vi "Main.vi"() -> ()   [LabVIEW 2022 SP3]
panel:
  in  "Number 8":dbl
  out "Result 4":dbl
  in  "Number 7":dbl
  in  "Number 6":dbl
  out "Result 3":dbl
  in  "Number 5":dbl
  in  "Number 4":dbl
  out "Result 2":dbl
  in  "Number 3":dbl
  in  "Number 2":dbl
  in  "Ending！":bool
  out "Result 1":dbl
  in  "Number 1":dbl
  # "Calculation 1——Simple"
  # "Add"
  # "+"
  # "="
  # "Subtract"
  # "-"
  # "="
  # "Multiple"
  # "*"
  # "="
  # "Divide"
  # "/"
  # "="
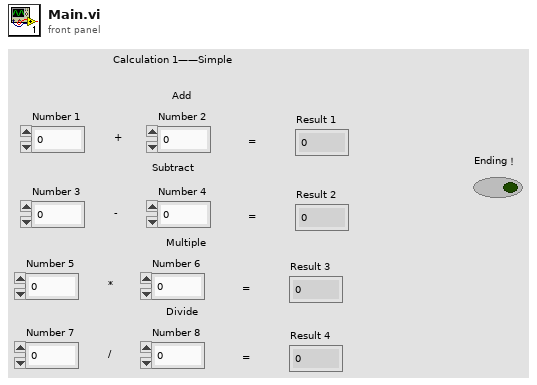
[diagram p1: front panel]
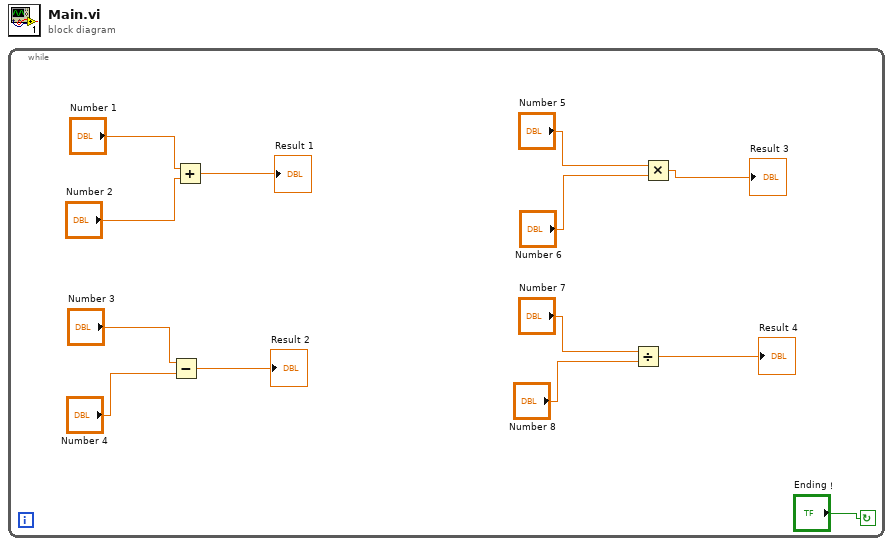
[diagram p0: block diagram]
diagram:
  n1 = while {
    stop <- "Ending！" continue-if-true
    n2 = Subtract(x="Number 3", y="Number 4") -> (x-y=→"Result 2":dbl)
    n3 = Add(x="Number 1", y="Number 2") -> (x+y=→"Result 1":dbl)
    n4 = Divide(x="Number 7", y="Number 8") -> (x/y=→"Result 4":dbl)
    n5 = Multiply(x="Number 5", y="Number 6") -> (x*y=→"Result 3":dbl)
  }
